vi "img.remapMarkerValues.vi"(7 "min intervals":dbl=4.0 caption="min intervals (4)", 10 "colours in":u32[](array[numeric]), 11 "marker values in":dbl[](array[numeric])) -> (2 "colours out":u32[](array[numeric]), 3 "marker values out":dbl[](array[numeric]), 5 "interval":dbl)   [LabVIEW 2020]
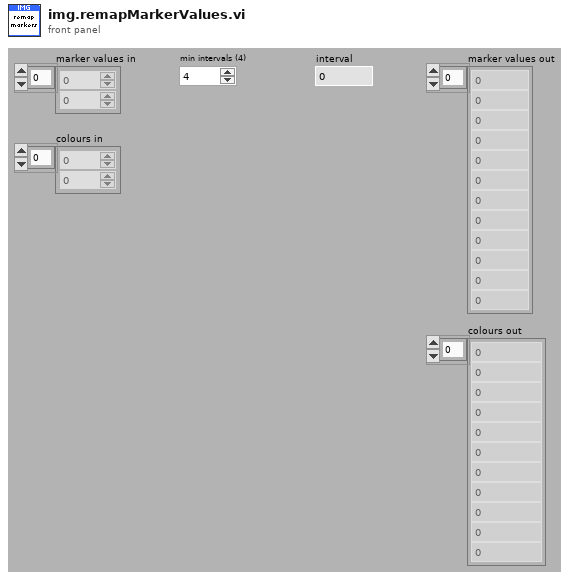
[diagram p1: front panel]
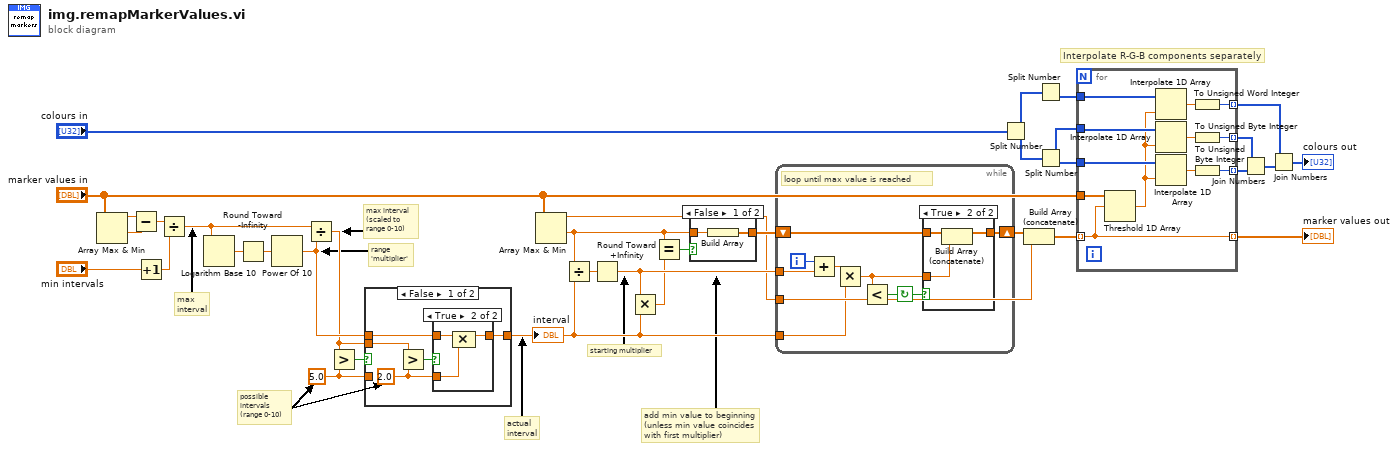
[diagram p0: block diagram]
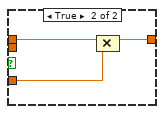
[diagram p5: hidden frame]
diagram:
  w34 = 5.0 ("y")
  # "Interpolate R-G-B components separately"
  # "add min value to beginning\n(unless min value coincides \nwith first multiplier)"
  # "starting multiplier"
  # "actual \ninterval"
  # "max \ninterval"
  # "range \n'multiplier'"
  # "max interval\n(scaled to\nrange 0-10)"
  # "possible\nintervals\n(range 0-10)"
  n1 = Array Max & Min(array="marker values in") -> (max value=w25:dbl, min value=w26:dbl)  [unwired: 2 out]
  n2 = Subtract(x=w25, y=w26) -> (x-y=w27:dbl)
  n3 = Increment(x="min intervals") -> (x+1=w28:dbl)
  n4 = Divide(x=w27, y=w28) -> (x/y=w31:dbl)
  n5 = Logarithm Base 10(1:w31) -> (0:w30:dbl)
  n6 = Round Toward -Infinity(1:w30) -> (0:w29:dbl)
  n7 = Power Of 10(x=w29) -> (10^x=w35:dbl)
  n8 = Divide(x=w31, y=w35) -> (x/y=w33:dbl)
  n9 = Greater?(x=w33, y=w34) -> (0:w32:bool)
  n10 = case shown="False" w32 {
    tunnel: w33 -> [w40 _]
    tunnel: w34 -> [_ w47]
    tunnel: w35 -> [w37 w46]
    tunnel: [w36 w45] -> w20
    frame False {
      w38 = 2.0 ("y")
      n11 = Greater?(x=w40, y=w38) -> (0:w39:bool)
      n12 = case shown="True" w39 {
        tunnel: w38 -> [_ w43]
        tunnel: w37 -> [w41 w44]
        tunnel: [w41 w42] -> w36
        frame False {
        }
        frame True {
          n13 = Compound Arithmetic op=MULTIPLY(w44, w43) -> (w42:dbl)
        }
      }
    }
    frame True {
      n14 = Compound Arithmetic op=MULTIPLY(w46, w47) -> (w45:dbl)
    }
  }
  "interval" <- w20
  n15 = Array Max & Min(array="marker values in") -> (max value=w15:dbl, min value=w18:dbl)  [unwired: 2 out]
  n16 = Divide(x=w18, y=w20) -> (x/y=w23:dbl)
  n17 = Round Toward +Infinity(x=w23) -> (ceil(x): smallest int >= x=w21:dbl)
  n18 = Multiply(x=w21, y=w20) -> (x*y=w19:dbl)
  n19 = Equal?(x=w18, y=w19) -> (x = y?=w17:bool)
  n20 = case shown="False" w17 {
    tunnel: w18 -> [w49 _]
    tunnel: [w48 _] -> w22
    frame False {
      n21 = Build Array(w49) -> (w48:dbl[])
    }
    frame True {
    }
  }
  n22 = while {
    tunnel: w21 -> [w51]
    tunnel: w20 -> [w58]
    shift-right: [w56] -> w16
    shift-left: w22 -> [w57]
    tunnel: w15 -> [w55]
    i -> [w52]
    stop <- w54 continue-if-true
    # "loop until max value is reached"
    n23 = Add(x=w52, y=w51) -> (x+y=w50:dbl)
    n24 = Multiply(x=w50, y=w58) -> (x*y=w53:dbl)
    n25 = Less?(x=w53, y=w55) -> (x < y?=w54:bool)
    n26 = case shown="True" w54 {
      tunnel: w57 -> [w59 w62]
      tunnel: [w59 w61] -> w56
      tunnel: w53 -> [_ w60]
      frame False {
      }
      frame True {
        n27 = Build Array (concatenate)(w62, w60) -> (w61:dbl[])
      }
    }
  }
  n28 = Split Number(x="colours in") -> (hi(x)=w7:u16[], lo(x)=w10:u16[])
  n29 = Build Array (concatenate)(w16, w15) -> (w14:dbl[])
  n30 = Split Number(x=w7) -> (lo(x)=w6:u8[])  [unwired: 1 out]
  n31 = Split Number(x=w10) -> (hi(x)=w8:u8[], lo(x)=w9:u8[])
  n32 = for {
    tunnel: w14 -> [w73] mode=indexing
    tunnel: [w73] -> w13 mode=indexing
    tunnel: w9 -> [w72]
    tunnel: "marker values in" -> [w74]
    tunnel: [w70] -> w5 mode=indexing
    tunnel: w8 -> [w67]
    tunnel: w6 -> [w65]
    tunnel: [w64] -> w2 mode=indexing
    tunnel: [w63] -> w1 mode=indexing
    n33 = Threshold 1D Array(2:w73, 3:w74) -> (0:w66:dbl)  [unwired: 1 out]
    n34 = Interpolate 1D Array(1:w66, 2:w65) -> (0:w69:dbl)
    n35 = Interpolate 1D Array(1:w66, 2:w67) -> (0:w68:dbl)
    n36 = Interpolate 1D Array(1:w66, 2:w72) -> (0:w71:dbl)
    n37 = To Unsigned Word Integer(number=w69) -> (unsigned 16bit integer=w64:u16)
    n38 = To Unsigned Byte Integer(number=w68) -> (unsigned 8bit integer=w63:u8)
    n39 = To Unsigned Byte Integer(number=w71) -> (unsigned 8bit integer=w70:u8)
  }
  "marker values out" <- w13
  n40 = Join Numbers(hi=w1, lo=w5) -> ((hi.lo)=w4:u16[])
  n41 = Join Numbers(hi=w2, lo=w4) -> ((hi.lo)=→"colours out":u32[])
